vi "Convert U16 Array to String.vi"(11 "U16 array":u16[](array[numeric])) -> (3 "string":string)   [LabVIEW 2021, in "NI Session Management V1 Client.lvlib" / "Session Reservation.lvclass"]
uses:
  Session Reservation.lvclass
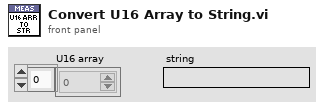
[diagram p1: front panel]
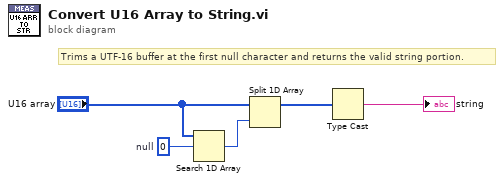
[diagram p0: block diagram]
diagram:
  w4 = u16 0  # null
  # "Trims a UTF-16 buffer at the first null character and returns the valid string portion."
  n1 = Search 1D Array(1D array="U16 array", element=w4) -> (index of element=w5:i32)  [unwired: 1 in]
  n2 = Split 1D Array(array="U16 array", index=w5) -> (first subarray=w1:u16[])  [unwired: 1 out]
  n3 = Type Cast(x=w1) -> (*(type *) &x=→"string":string)  [unwired: 1 in]
